vi "ConvertDistToDot.vi"(8 "错误输入（无错误）":errorcluster, 9 "当前零位偏移":i32, 10 "需要转换的距离":sgl, 11 "当前通道":u8) -> (0 "错误输出":errorcluster, 3 "返回值":u32)   [LabVIEW 2014]
uses:
  X86Dll/ZXUTConfigMgr.dll
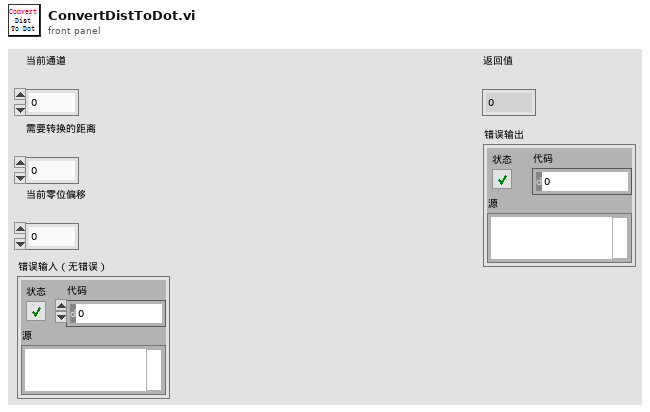
[diagram p1: front panel]
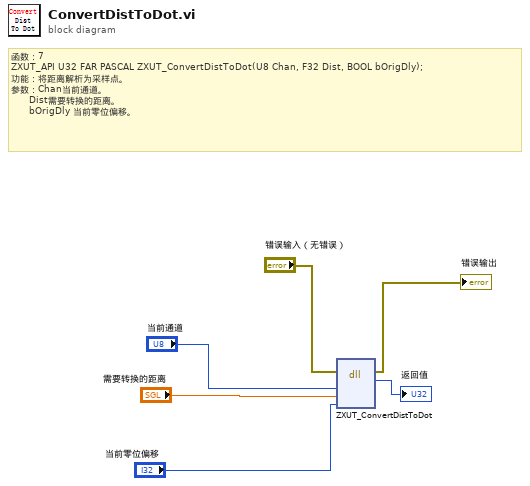
[diagram p0: block diagram]
diagram:
  # "函数：7\nZXUT_API U32\tFAR PASCAL ZXUT_ConvertDistToDot(U8 Chan, F32 Dist, BOOL bOrigDly);\n功能：将距离解析为采样点。\n参数：Chan当前通道。\n      Dist需要转换的距离。\n      bOrigDly 当前零位偏移。"
  n1 = dll-call lib="D:/Software/Utrasonic on-line monitoring/X86Dll/ZXUTConfigMgr.dll" fn="ZXUT_ConvertDistToDot"(error in="错误输入（无错误）", "Chan"="当前通道", "Dist"="需要转换的距离", "bOrigDly"="当前零位偏移") -> (error out=→"错误输出":errorcluster, "返回值"=→"返回值":u32)  [unwired: 5 in, 1 out]
